vi "Operator.vi"() -> ()   [LabVIEW 2023]
panel:
  in  "stop":bool
  out "Arkuszowa":bool
  out "Skalnicowa":bool
  out "Zabraniecka":bool
  out "Okopowa":bool
  out "Zwiry_i_Wigury":bool
  out "AirportCH":bool
  out "Wilanowska":bool
  out "Polczynska":bool
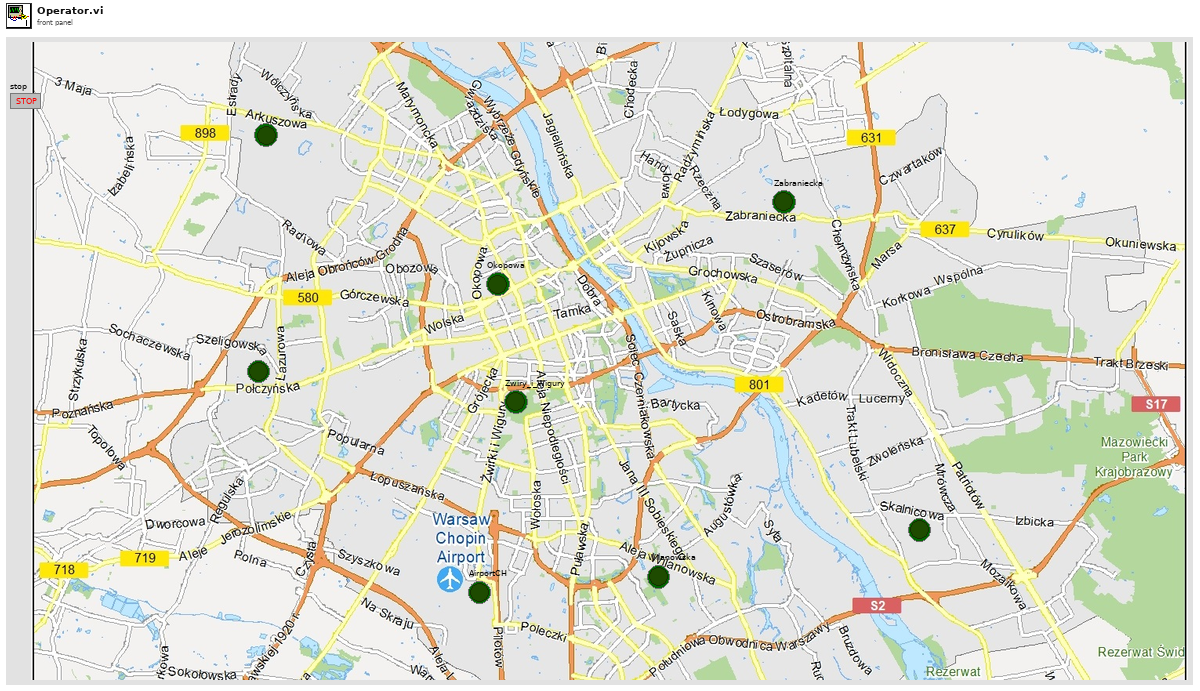
[diagram p1: front panel]
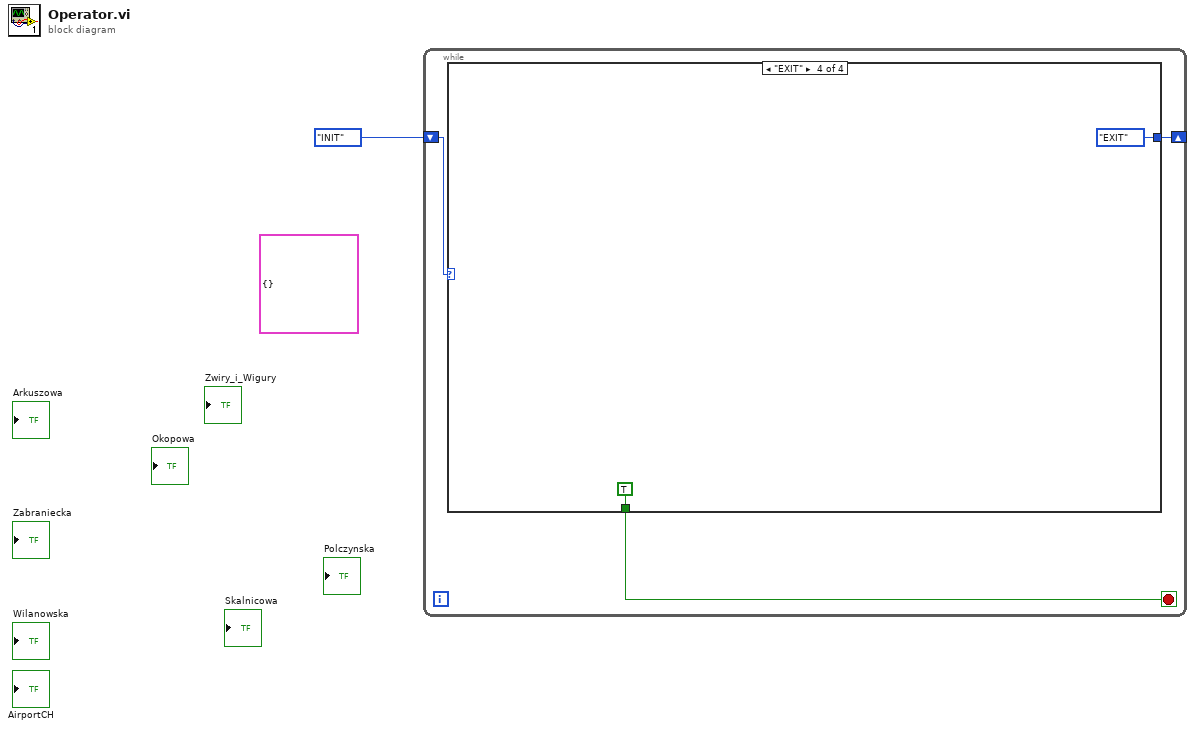
[diagram p0: block diagram]
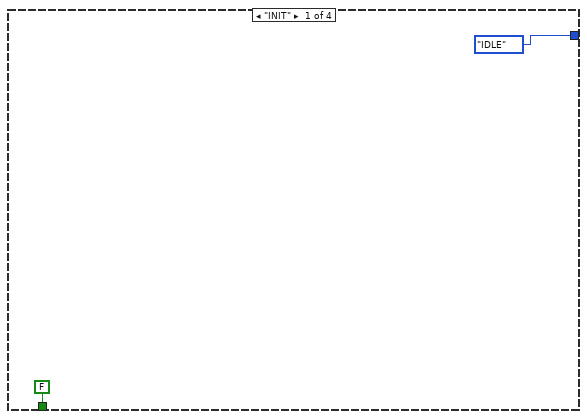
[diagram p2: hidden frame]
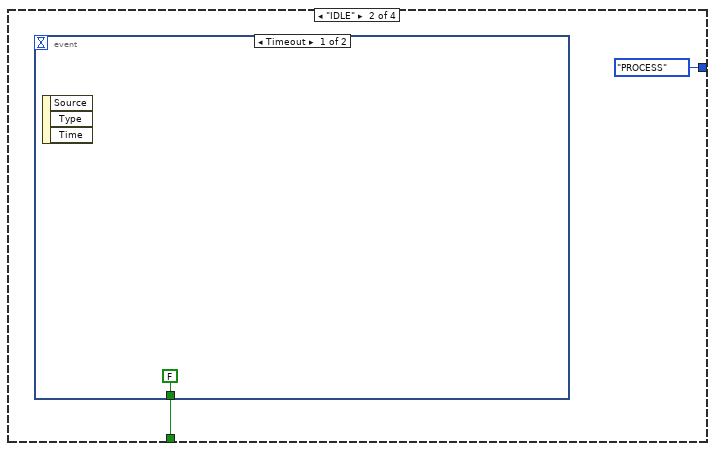
[diagram p3: hidden frame]
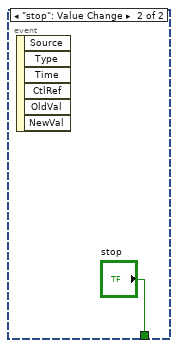
[diagram p4: hidden frame]
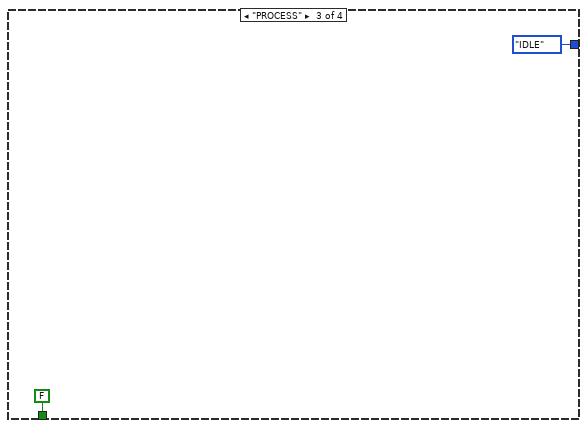
[diagram p5: hidden frame]
diagram:
  (unwired) cluster{} {}
  n1 = while {
    shift-right: [w3] -> _
    shift-left: enum16{"INIT", "IDLE", "PROCESS", "EXIT"}."INIT" -> [w4]
    stop <- w2 stop-if-true
    n2 = case shown="\"EXIT\"" w4 {
      tunnel: [enum16{"INIT", "IDLE", "PROCESS", "EXIT"}."IDLE" enum16{"INIT", "IDLE", "PROCESS", "EXIT"}."PROCESS" enum16{"INIT", "IDLE", "PROCESS", "EXIT"}."IDLE" enum16{"INIT", "IDLE", "PROCESS", "EXIT"}."EXIT"] -> w3
      tunnel: [FALSE ("stop") w7 FALSE ("stop") TRUE ("stop")] -> w2
      frame "INIT" {
      }
      frame "IDLE" {
        n3 = event shown="[0] Timeout" {
          selector: _ -> [_ _]
          dyn-events: _ -> [_ _]
          timeout: _ -> [_ _]
          tunnel: [FALSE ("stop") "stop"] -> w7
          event Timeout {
            n4 = event-data() -> ()  [unwired: 1 in, 3 out]
          }
          event "stop": Value Change {
            n5 = event-data() -> ()  [unwired: 1 in, 6 out]
          }
        }
      }
      frame "PROCESS" {
      }
      frame "EXIT" {
      }
    }
  }
